vi "Calculate Loss (Available Gain Definition).vi"(5 "Termination":cdb[](array[numeric]), 6 "error in (no error)":errorcluster, 9 "2-port S-parameters":cdb[][](array[numeric])) -> (0 "error out":errorcluster, 3 "Loss":dbl[](array[numeric]))   [LabVIEW 2023, in "NI_HFNetworkAnalysis.lvlib"]
doc: "Calculates the mismatch loss of a 2-port network at different frequencies when it is terminated by the specified termination.\n\nMismatch loss is calculated using <b>available gain definition</b>.\n\nThe network is defined by 2-port S-parameters <b>(S11,S12,S21,S22)</b> at different frequencies and the termination is described by its reflection factor at those frequencies.\n\n<b>Known Limitations</b>\nOnly 2-port networks are supported."
uses:
  NI_HFNetworkAnalysis.lvlib
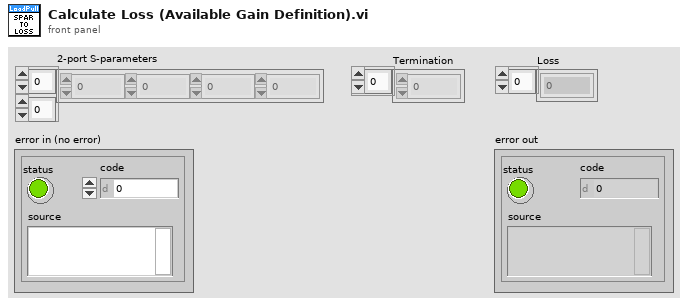
[diagram p1: front panel]
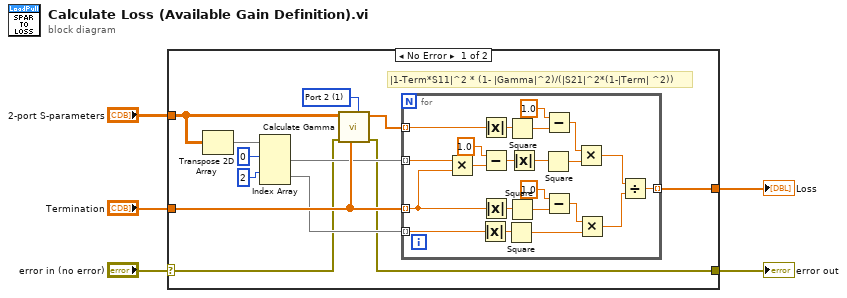
[diagram p0: block diagram]
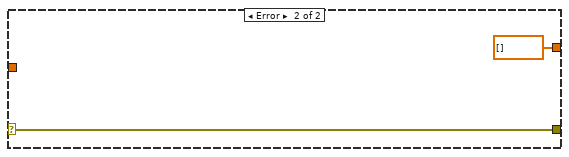
[diagram p2: hidden frame]
diagram:
  n1 = case shown="No Error" "error in (no error)" {
    selector: "error in (no error)" -> [w7 w41]
    tunnel: [w17 dbl[] []] -> w5
    tunnel: "Termination" -> [w15 _]
    tunnel: "2-port S-parameters" -> [w8 _]
    tunnel: [w6 w41] -> w1
    frame No Error {
      w11 = u16 1 items=["Port 1", "Port 2"] ("Port")
      # "|1-Term*S11|^2 * (1- |Gamma|^2)/(|S21|^2*(1-|Term| ^2))"
      n2 = Transpose 2D Array(2D array=w8) -> (transposed array=w14:cdb[][])
      n3 = Index Array(array=w14, index (row) #1=0 ("index (row)"), index (row) #2=2 ("index (row)")) -> (element #1=w13:cdb[], element #2=w12:cdb[])  [unwired: 2 in]
      n4 = call "Calculate Gamma.vi"("Port (Port 1)"=w11, "Termination"=w15, "error in (no error)"=w7, "2-port S-parameters"=w8) -> ("error out"=w6:errorcluster, "Gamma"=w16:cdb[])  [unwired: 4 in]
      n5 = for {
        tunnel: [w18] -> w17 mode=indexing
        tunnel: w16 -> [w31] mode=indexing
        tunnel: w13 -> [w28] mode=indexing
        tunnel: w12 -> [w35] mode=indexing
        tunnel: w15 -> [w27] mode=indexing
        n6 = Multiply(x=w28, y=w27) -> (x*y=w25:cdb)
        n7 = Absolute Value(x=w35) -> (abs(x)=w36:dbl)
        n8 = Absolute Value(x=w31) -> (abs(x)=w30:dbl)
        n9 = Subtract(x=1.0, y=w25) -> (x-y=w24:cdb)
        n10 = Absolute Value(x=w27) -> (abs(x)=w38:dbl)
        n11 = Square(x=w36) -> (x^2=w34:dbl)
        n12 = Square(x=w30) -> (x^2=w29:dbl)
        n13 = Square(x=w38) -> (x^2=w37:dbl)
        n14 = Absolute Value(x=w24) -> (abs(x)=w23:dbl)
        n15 = Square(x=w23) -> (x^2=w22:dbl)
        n16 = Subtract(x=1.0, y=w29) -> (x-y=w21:dbl)
        n17 = Subtract(x=1.0, y=w37) -> (x-y=w33:dbl)
        n18 = Multiply(x=w21, y=w22) -> (x*y=w20:dbl)
        n19 = Multiply(x=w33, y=w34) -> (x*y=w19:dbl)
        n20 = Divide(x=w20, y=w19) -> (x/y=w18:dbl)
      }
    }
    frame Error {
    }
  }
  "Loss" <- w5
  "error out" <- w1
